vi "Single Pulse Generation.vi"   [LabVIEW 2009]
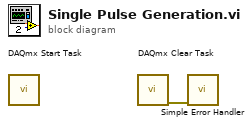
[diagram p0: block diagram]
diagram:
  n1 = call <vilib>:"DAQmx Start Task.vi"() -> ()  [unwired: 14 in, 2 out]
  n2 = call <vilib>:"DAQmx Clear Task.vi"() -> ("error out"=w1:errorcluster)  [unwired: 15 in]
  n3 = call <vilib>:"Simple Error Handler.vi"("error in (no error)"=w1) -> ()  [unwired: 4 in, 5 out]
